vi "Turret Mangement.vi"(0 "Servo":T1={"DeviceStatus"={"status"=FALSE, "code"=0, "source"=""}, "Digital Module"=enum."Digital Module 1", "PWM Channel"=enum."Invalid", "DeadBand"={"Name"="", "maxPositivePwm"=0, "minPositivePwm"=0, "centerPwm"=0, "maxNegativePwm"=0, "minNegativePwm"=0, "angularRange"=0}}, 1 "Straigthener":dbl, 2 "DashBoard Info":T5, 3 "Left":T6, 4 "AutoSearch":bool, 5 "Right":T6, 8 "Turret Override Input":dbl, 9 "Pitch Current":dbl, 10 "Turret Override":bool, 11 "Sync cam&cannon":bool) -> (12 "Fixed Distance[m]":dbl, 14 "Fixed Height[m]":dbl, 16 "Locked On Target":bool, 17 "Fixed Angle[deg]":dbl, 18 "Servo":i32, 19 "Turret":dbl)   [LabVIEW 2011]
uses:
  <vilib>/Rock Robotics/WPI/DigitalInput/WPI_DigitalInputDevRef.ctl
  <vilib>/Rock Robotics/SystemInterfaces/DIO/FPGA_DIOChannel.ctl
  <vilib>/Rock Robotics/SystemInterfaces/Typedef/FPGA_TypedefDigitalModule.ctl
  <vilib>/Rock Robotics/WPI/PWM/Servo/WPI_ServoDeviceRef.ctl
  <vilib>/Rock Robotics/SystemInterfaces/DIO/FPGA_DIOPWMChannel.ctl
  <vilib>/Rock Robotics/WPI/PWM/WPI_PWMDeadband.ctl
  cupStateGlobal.vi
  <vilib>/ptbypt/NI_PtbyPt.lvlib
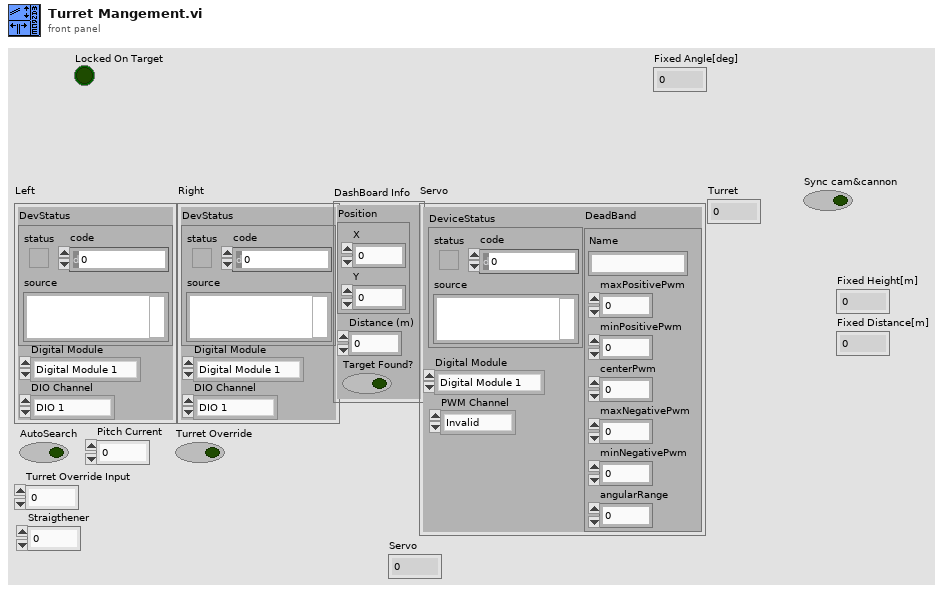
[diagram p1: front panel]
types:
  T1 = typedef "WPI_ServoDeviceRef.ctl" = cluster{"DeviceStatus":errorcluster, "Digital Module":T2, "PWM Channel":T3, "DeadBand":T4}
  T2 = typedef "FPGA_TypedefDigitalModule.ctl" = enum16{"Digital Module 1", "Digital Module 2"}
  T3 = typedef "FPGA_DIOPWMChannel.ctl" = enum8{"PWM 1", "PWM 2", "PWM 3", "PWM 4", "PWM 5", "PWM 6", "PWM 7", "PWM 8", "PWM 9", "PWM 10", "Invalid"}
  T4 = typedef "WPI_PWMDeadband.ctl" = cluster{"Name":string, "maxPositivePwm":i32, "minPositivePwm":i32, "centerPwm":i32, "maxNegativePwm":i32, "minNegativePwm":i32, "angularRange":u16}
  T5 = cluster{"Position":cluster{"X":dbl, "Y":dbl}, "Distance (m)":dbl, "Target Found?":bool}
  T6 = typedef "WPI_DigitalInputDevRef.ctl" = cluster{"DevStatus":errorcluster, "DIO Channel":T7, "Digital Module":T2}
  T7 = typedef "FPGA_DIOChannel.ctl" = enum8{"DIO 1", "DIO 2", "DIO 3", "DIO 4", "DIO 5", "DIO 6", "DIO 7", "DIO 8", "DIO 9", "DIO 10", "DIO 11", "DIO 12", "DIO 13", "DIO 14", "Invalid"}
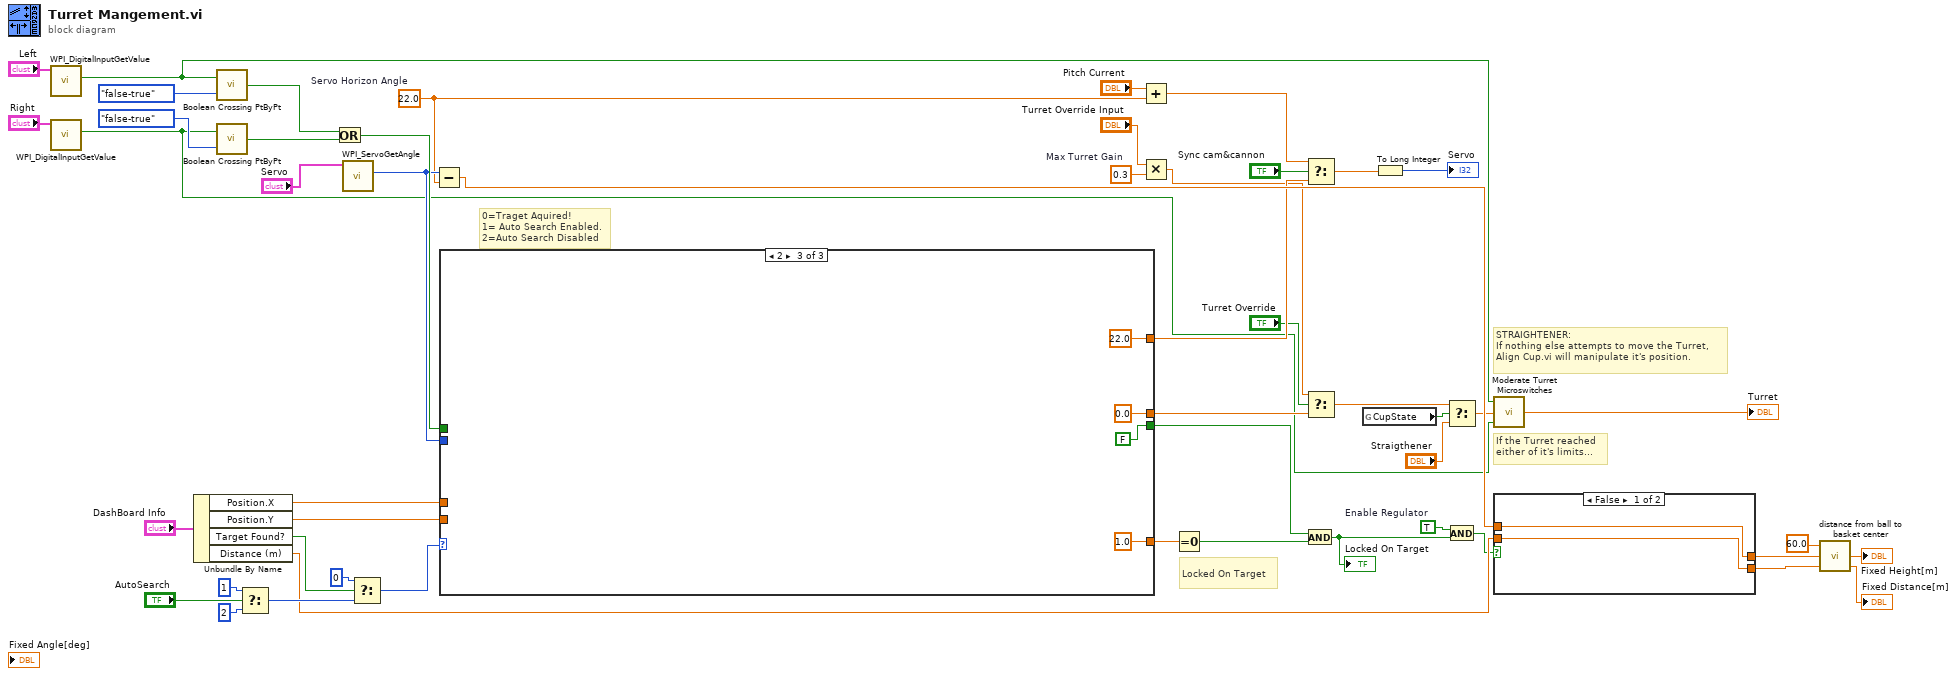
[diagram p0: block diagram]
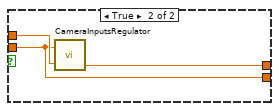
[diagram p2: hidden frame]
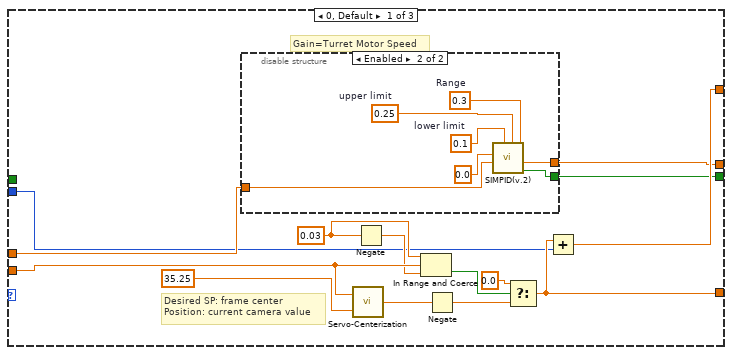
[diagram p3: hidden frame]
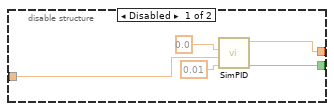
[diagram p4: hidden frame]
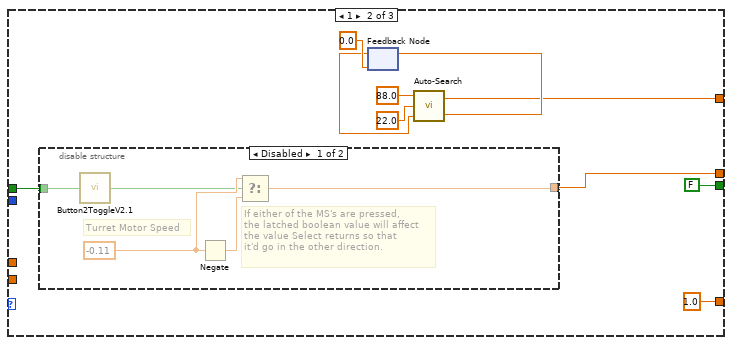
[diagram p5: hidden frame]
diagram:
  w3 = TRUE  # Enable Regulator
  w20 = 0.3  # Max Turret Gain
  w26 = 22.0  # Servo Horizon Angle
  # "If the Turret reached \neither of it's limits..."
  # "0=Traget Aquired!\n1= Auto Search Enabled.\n2=Auto Search Disabled"
  # "STRAIGHTENER:\nIf nothing else attempts to move the Turret,\nAlign Cup.vi will manipulate it's position."
  # "Locked On Target"
  n1 = call <vilib>:"WPI_DigitalInputGetValue.vi"("DigitalInputDevRef"="Left") -> ("Value"=w12:bool)  [unwired: 8 in, 2 out]
  n2 = call <vilib>:"WPI_DigitalInputGetValue.vi"("DigitalInputDevRef"="Right") -> ("Value"=w13:bool)  [unwired: 8 in, 2 out]
  n3 = Unbundle By Name("DashBoard Info") -> ("Position.X"=w37:dbl, "Position.Y"=w36:dbl, "Target Found?"=w42:bool, "Distance (m)"=w9:dbl)
  n4 = call <vilib>:"Boolean Crossing PtByPt.vi"("direction"=enum16{"either", "false-true", "true-false"}."false-true", "input"=w12) -> ("crossing"=w47:bool)  [unwired: 1 in]
  n5 = call <vilib>:"Boolean Crossing PtByPt.vi"("direction"=enum16{"either", "false-true", "true-false"}."false-true", "input"=w13) -> ("crossing"=w14:bool)  [unwired: 1 in]
  n6 = Select(t=1 ("Position.X"), s="AutoSearch", f=2 ("Position.X")) -> (s? t:f=w43:i32)
  n7 = Or(x=w47, y=w14) -> (x .or. y?=w38:bool)
  n8 = call <vilib>:"WPI_ServoGetAngle.vi"("ServoDeviceRef"="Servo") -> ("Angle"=w33:u16)  [unwired: 7 in, 2 out]
  n9 = Select(t=0 ("Position.X"), s=w42, f=w43) -> (s? t:f=w39:i32)
  n10 = Subtract(x=w33, y=w26) -> (x-y=w34:dbl)
  n11 = case shown="2" w39 {
    tunnel: [w57 w82 22.0 ("Servo Angle")] -> w27
    tunnel: w36 -> [w60 _ _]
    tunnel: w37 -> [w55 _ _]
    tunnel: [w56 1.0 ("Rounded Error") 1.0 ("Rounded Error")] -> w30
    tunnel: [w54 FALSE ("On Target") FALSE ("On Target")] -> w31
    tunnel: [w53 w78 0.0 ("t")] -> w17
    tunnel: w38 -> [_ w79 _]
    tunnel: w33 -> [w52 _ _]
    frame 0, Default {
      w59 = 0.03 ("lower limit")
      # "Desired SP: frame center\nPosition: current camera value"
      # "Gain=Turret Motor Speed"
      n12 = disable-structure shown="Enabled" {
        disable-tunnel: w55 -> [w70 w73]
        disable-tunnel: [w67 w71] -> w54
        disable-tunnel: [w66 w72] -> w53
        frame Disabled {
          n13 = call "SimPID.vi"("Range"=0.01, "Position"=w70, "Set Point"=0.0) -> ("On Target"=w67:bool, "result"=w66:dbl)  [unwired: 6 in]
        }
        frame Enabled {
          w76 = 0.3  # Range
          w75 = 0.25  # upper limit
          w74 = 0.1  # lower limit
          n14 = call "SIMPID(v.2).vi"("Range"=w76, "upper limit"=w75, "lower limit"=w74, "Current Point"=w73, "Set Point"=0.0) -> ("On Target"=w71:bool, "result"=w72:dbl)  [unwired: 5 in]
        }
      }
      n15 = call "Servo-Centerization.vi"("Camera Angle"=35.25 ("HALF Cam angle constant"), "Cartez"=w60) -> ("Rounded Error"=w64:dbl)
      n16 = Negate(x=w59) -> (-x=w58:dbl)
      n17 = In Range and Coerce(upper limit=w59, x=w60, lower limit=w58) -> (In Range?=w61:bool)  [unwired: 1 out]
      n18 = Negate(x=w64) -> (-x=w65:dbl)
      n19 = Select(t=0.0 ("f"), s=w61, f=w65) -> (s? t:f=w56:dbl)
      n20 = Add(x=w56, y=w52) -> (x+y=w57:dbl)
    }
    frame 1 {
      n21 = disable-structure shown="Disabled" {
        disable-tunnel: w79 -> [w89 _]
        disable-tunnel: [w90 _] -> w78
        frame Disabled {
          w92 = -0.11 ("t")
          # "If either of the MS's are pressed,\nthe latched boolean value will affect\nthe value Select returns so that\nit'd go in the other direction."
          # "Turret Motor Speed"
          n22 = call "Button2ToggleV2.1.vi"("a"=w89) -> ("Result(clone)"=w88:bool)
          n23 = Negate(x=w92) -> (-x=w91:dbl)
          n24 = Select(t=w92, s=w88, f=w91) -> (s? t:f=w90:dbl)
        }
        frame Enabled {
        }
      }
      n25 = feedback #1(0.0 ("counter")) -> (w86:dbl)
      n26 = call "Auto-Search.vi"("Counter\\Timer"=w86, "Low Angle Edge"=22.0, "High Angle Edge"=88.0) -> ("counter"=w85:dbl, "Servo Angle"=w82:dbl)
      n27 = feedback-in #1(w85) -> ()
    }
    frame 2 {
    }
  }
  n28 = Add(x="Pitch Current", y=w26) -> (x+y=w28:dbl)
  n29 = Multiply(x="Turret Override Input", y=w20) -> (x*y=w18:dbl)
  n30 = Equal To 0?(x=w30) -> (x = 0?=w32:bool)
  n31 = And(x=w31, y=w32) -> (x .and. y?=w4:bool)
  "Locked On Target" <- w4
  n32 = Select(t=w28, s="Sync cam&cannon", f=w27) -> (s? t:f=w24:dbl)
  n33 = Select(t=w18, s="Turret Override", f=w17) -> (s? t:f=w22:dbl)
  n34 = global read "cupStateGlobal.vi" "CupState"() -> (w10:bool)
  n35 = To Long Integer(number=w24) -> (32bit integer=→"Servo":i32)
  n36 = Select(t=w22, s=w10, f="Straigthener") -> (s? t:f=w16:dbl)
  n37 = And(x=w3, y=w4) -> (x .and. y?=w2:bool)
  n38 = call "Moderate Turret Microswitches.vi"("TurretRightMS"=w13, "Input"=w16, "TurretLeftMS"=w12) -> ("Output"=→"Turret":dbl)
  n39 = case shown="False" w2 {
    tunnel: w34 -> [w98 w101]
    tunnel: w9 -> [w97 w99]
    tunnel: [w98 w100] -> w8
    tunnel: [w97 w99] -> w1
    frame False {
    }
    frame True {
      n40 = call "CameraInputsRegulator.vi"("Distance[m]"=w99, "Angle(servo)"=w101) -> ("Fixed Angle[deg]"=w100:dbl)  [unwired: 2 out]
    }
  }
  n41 = call "distance from ball to basket center.vi"("d"=w1, "alpha"=w8, "theta"=60.0) -> ("horizontal D2T [m]"=→"Fixed Distance[m]":dbl, "Vertical D2T [m]"=→"Fixed Height[m]":dbl)  [unwired: 1 out]
